vi "server.vi"() -> ()   [LabVIEW 2014]
panel:
  out "data received from client":string
  in  "address in client":string
  in  "function code":string
  in  "data to be written":string
  in  "client id":string
  in  "unicast":bool
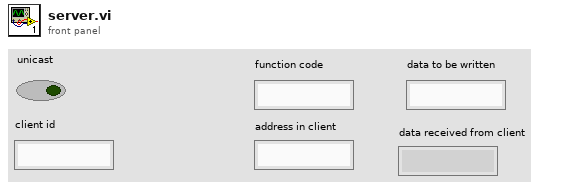
[diagram p1: front panel]
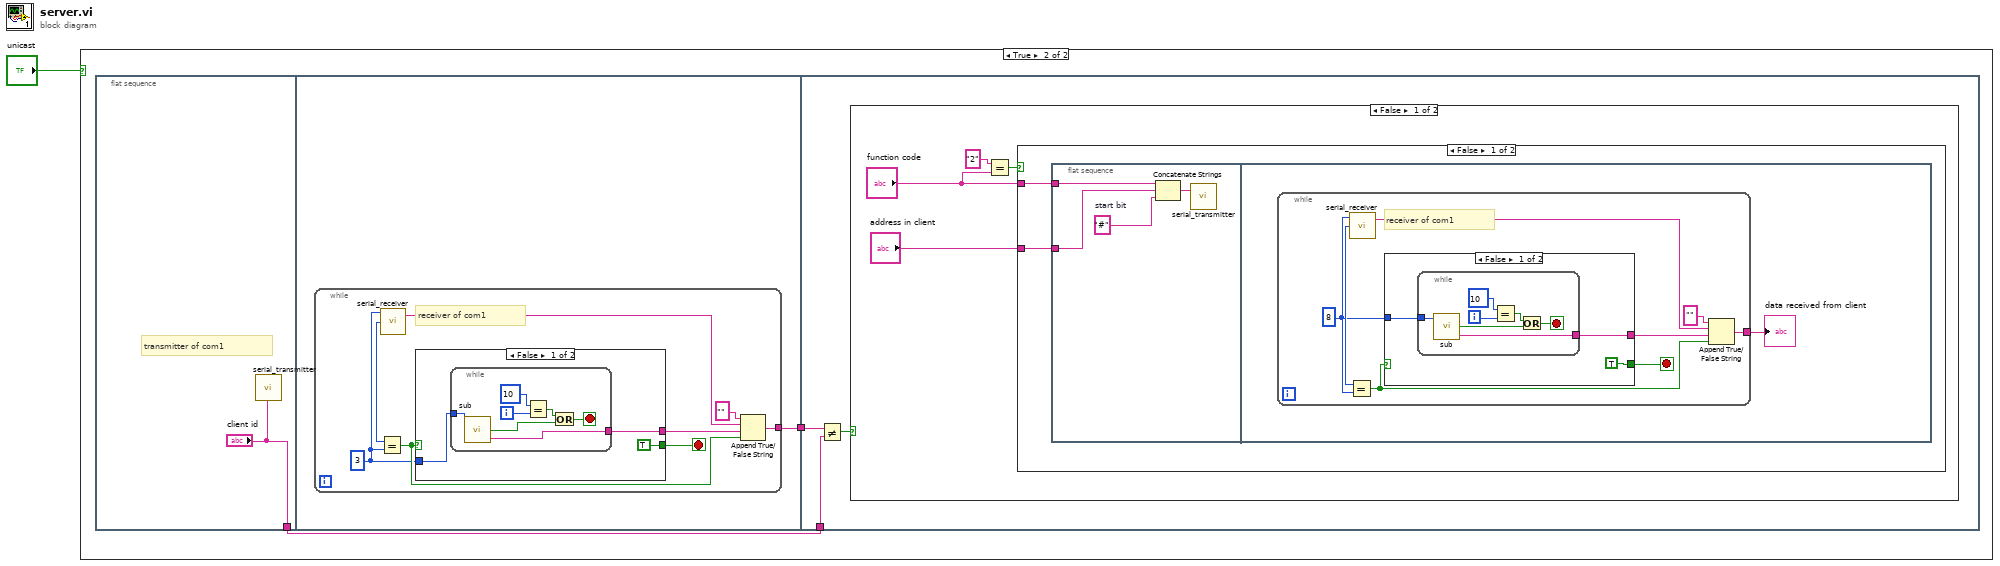
[diagram p0: block diagram]
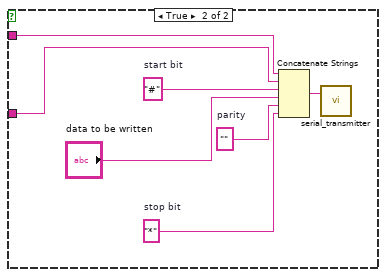
[diagram p5: hidden frame]
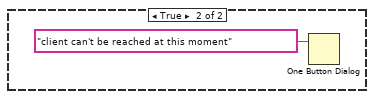
[diagram p6: hidden frame]
diagram:
  n1 = case shown="True" "unicast" {
    frame False {
    }
    frame True {
      n2 = flat-sequence {
        tunnel: ["client id"] -> w2
        tunnel: [w5] -> w3
        tunnel: w3 -> [w27]
        tunnel: w2 -> [w26]
        frame #0 {
          # "transmitter of com1"
          n3 = call "serial_transmitter.vi"("write buffer"="client id") -> ()  [unwired: 1 in, 2 out]
        }
        frame #1 {
          n4 = while {
            tunnel: [w7] -> w5
            stop <- w12 stop-if-true
            w6 = u32 3 ("byte count")
            # "receiver of com1"
            n5 = call "serial_receiver.vi"("byte count"=w6) -> ("read buffer"=w10:string, "return count"=w13:u32)  [unwired: 1 in, 1 out]
            n6 = Equal?(x=w13, y=w6) -> (x = y?=w8:bool)
            n7 = case shown="False" w8 {
              selector: w8 -> [_ w24]
              tunnel: [TRUE w24] -> w12
              tunnel: [w16 _] -> w9
              tunnel: w6 -> [w14 _]
              frame False {
                n8 = while {
                  tunnel: [w18] -> w16
                  tunnel: w14 -> [w17]
                  i -> [w23]
                  stop <- w20 stop-if-true
                  n9 = call "sub.vi"("byte count"=w17) -> ("read buffer"=w18:string, "x = y?"=w19:bool)
                  n10 = Equal?(x=10, y=w23) -> (x = y?=w21:bool)
                  n11 = Or(x=w21, y=w19) -> (x .or. y?=w20:bool)
                }
              }
              frame True {
              }
            }
            n12 = Append True/False String(1:w8, 2:w9, 3:w10, 4:"" ("string (\"\")")) -> (0:w7:string)
          }
        }
        frame #2 {
          n13 = Not Equal?(x=w27, y=w26) -> (x != y?=w25:bool)
          n14 = case shown="False" w25 {
            frame False {
              n15 = Equal?(x="2", y="function code") -> (x = y?=w29:bool)
              n16 = case shown="False" w29 {
                tunnel: "function code" -> [w33 w59]
                tunnel: "address in client" -> [w32 w58]
                frame False {
                  n17 = flat-sequence {
                    tunnel: w33 -> [w35]
                    tunnel: w32 -> [w34]
                    frame #0 {
                      w37 = "#"  # start bit
                      n18 = Concatenate Strings(w35, w34, w37) -> (w36:string)
                      n19 = call "serial_transmitter.vi"("write buffer"=w36) -> ()  [unwired: 1 in, 2 out]
                    }
                    frame #1 {
                      n20 = while {
                        tunnel: [w40] -> w38
                        stop <- w45 stop-if-true
                        w39 = u32 8 ("byte count")
                        # "receiver of com1"
                        n21 = call "serial_receiver.vi"("byte count"=w39) -> ("read buffer"=w43:string, "return count"=w46:u32)  [unwired: 1 in, 1 out]
                        n22 = Equal?(x=w46, y=w39) -> (x = y?=w41:bool)
                        n23 = case shown="False" w41 {
                          selector: w41 -> [_ w57]
                          tunnel: [TRUE w57] -> w45
                          tunnel: [w49 _] -> w42
                          tunnel: w39 -> [w47 _]
                          frame False {
                            n24 = while {
                              tunnel: [w51] -> w49
                              tunnel: w47 -> [w50]
                              i -> [w56]
                              stop <- w53 stop-if-true
                              n25 = call "sub.vi"("byte count"=w50) -> ("read buffer"=w51:string, "x = y?"=w52:bool)
                              n26 = Equal?(x=10, y=w56) -> (x = y?=w54:bool)
                              n27 = Or(x=w54, y=w52) -> (x .or. y?=w53:bool)
                            }
                          }
                          frame True {
                          }
                        }
                        n28 = Append True/False String(1:w41, 2:w42, 3:w43, 4:"" ("string (\"\")")) -> (0:w40:string)
                      }
                      "data received from client" <- w38
                    }
                  }
                }
                frame True {
                  w61 = "*"  # stop bit
                  w62 = ""  # parity
                  w63 = "#"  # start bit
                  n29 = Concatenate Strings(w59, w58, w63, "data to be written", w62, w61) -> (w60:string)
                  n30 = call "serial_transmitter.vi"("write buffer"=w60) -> ()  [unwired: 1 in, 2 out]
                }
              }
            }
            frame True {
              n31 = One Button Dialog(message="client can't be reached at this moment") -> ()  [unwired: 1 in, 1 out]
            }
          }
        }
      }
    }
  }
